vi "initialiseComPort.vi"(2 "error in (no error)":errorcluster, 3 "BK1823ACounter.lvclass":refnum<class "BK1823ACounter.lvclass">) -> (0 "error out":errorcluster, 1 "BK1823ACounter.lvclass 2":refnum<class "BK1823ACounter.lvclass">)   [LabVIEW 2011, in "Hardware.lvlib" / "frequencyCounters.lvlib" / "BK1823ACounter.lvclass"]
uses:
  BK1823ACounter.lvclass
  BK1823ACounter.lvclass/BK1823ACounter.ctl
  <vilib>/Instr/_visa.llb/VISA Configure Serial Port (Instr).vi
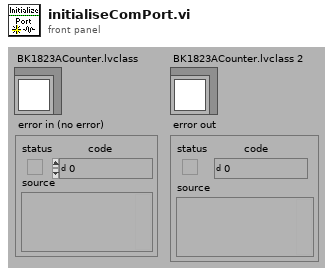
[diagram p1: front panel]
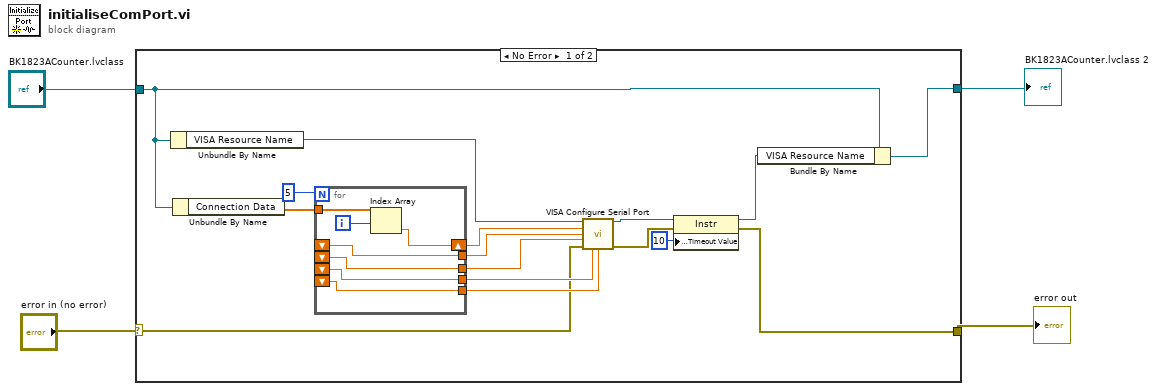
[diagram p0: block diagram]
diagram:
  n1 = case shown="No Error" "error in (no error)" {
    selector: "error in (no error)" -> [w12 w28]
    tunnel: "BK1823ACounter.lvclass" -> [w6 w29]
    tunnel: [w7 w28] -> w3
    tunnel: [w5 w29] -> w1
    frame No Error {
      n2 = Unbundle By Name(w6) -> ("VISA Resource Name"=w18:refnum<visa-resource-name>)
      n3 = Unbundle By Name(w6) -> ("Connection Data"=w19:dbl[])
      n4 = for {
        N: 5 -> [_]
        tunnel: w19 -> [w26]
        shift-right: [w25] -> w17
        shift-left: _ -> [w24]
        tunnel: [w24] -> w16
        shift-left: _ -> [w23]
        tunnel: [w23] -> w13
        shift-left: _ -> [w21]
        tunnel: [w21] -> w15
        shift-left: _ -> [w22]
        tunnel: [w22] -> w14
        i -> [w27]
        n5 = Index Array(array=w26, index=w27) -> (element=w25:dbl)
      }
      n6 = call-poly "VISA Configure Serial Port"("VISA resource name"=w18, "baud rate (9600)"=w17, "data bits (8)"=w16, "parity (0:none)"=w13, "error in (no error)"=w12, "stop bits (10: 1 bit)"=w15, "flow control (0:none)"=w14) -> ("VISA resource name out"=w10:refnum<visa-resource-name>, "error out"=w8:errorcluster)  [unwired: 7 in]
      n7 = property class="Instr"(reference=w10, error in=w8, "General Settings:Timeout Value"=u32 10) -> (reference out=w9:refnum<visa-resource-name>, error out=w7:errorcluster)
      n8 = Bundle By Name(cluster=w6, "VISA Resource Name"=w9) -> (w5:refnum<class "BK1823ACounter.lvclass">)
    }
    frame Error {
    }
  }
  "error out" <- w3
  "BK1823ACounter.lvclass 2" <- w1
